vi "EOL CAN_Get Key C70.vi"(11 "Seed message":u8[](array[numeric])=[6, 103, 1, 36, 34, 32, 31, 0] format="%x") -> (3 "Key":u32[](array[numeric]) format="%x")   [LabVIEW 2018]
panel:
  out "(hi.lo)":u32
  out "Seed":u32[](array[numeric])=[6, 103, 1, 36, 34, 32, 31, 0] format="%x"
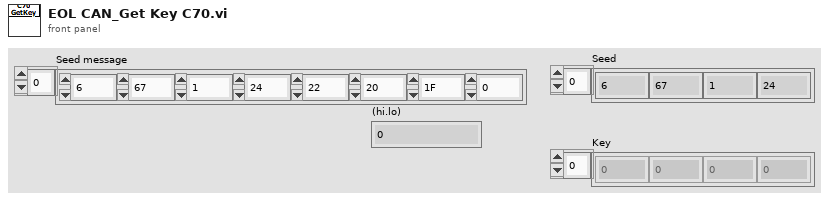
[diagram p1: front panel]
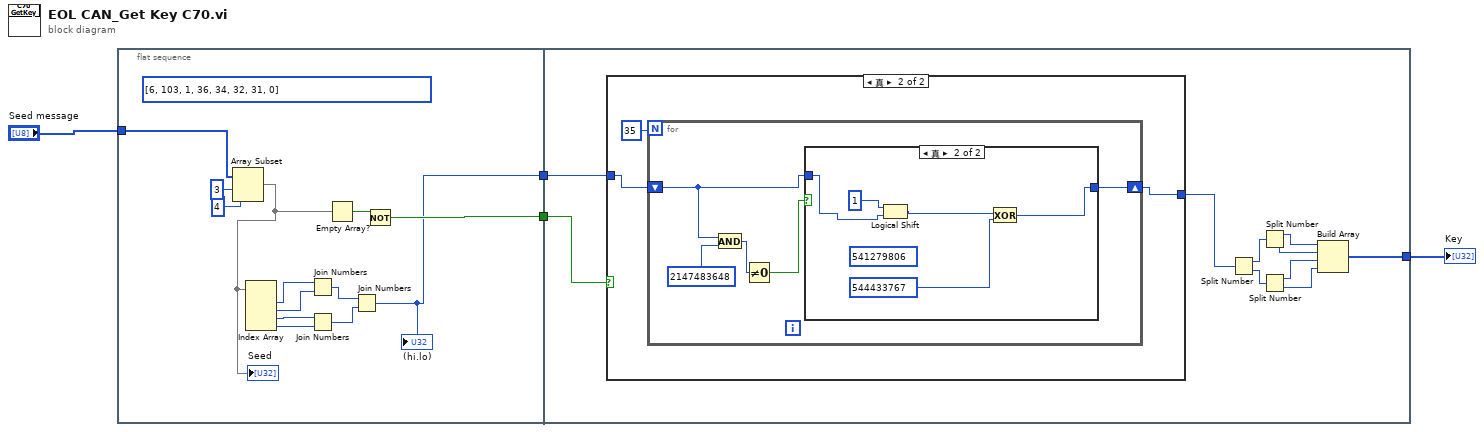
[diagram p0: block diagram]
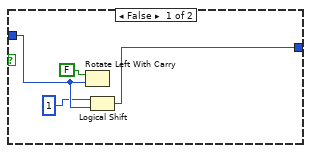
[diagram p3: hidden frame]
diagram:
  n1 = flat-sequence {
    tunnel: [w14] -> w4
    tunnel: [w7] -> w3
    tunnel: "Seed message" -> [w5]
    tunnel: w4 -> [w27]
    tunnel: w3 -> [w26]
    tunnel: [w18] -> w2
    frame #0 {
      (unwired) u8[] [6, 103, 1, 36, 34, 32, 31, 0] ("Transmit Data 2")
      n2 = Array Subset(array=w5, index=3 ("索引"), length=4 ("长度")) -> (w6:u8[])
      "Seed" <- w6
      n3 = Index Array(array=w6) -> (element #1=w13:u8, element #2=w12:u8, element #3=w11:u8, element #4=w10:u8)  [unwired: 4 in]
      n4 = Join Numbers(hi=w13, lo=w12) -> ((hi.lo)=w9:u16)
      n5 = Join Numbers(hi=w11, lo=w10) -> ((hi.lo)=w8:u16)
      n6 = Empty Array?(array=w6) -> (empty?=w15:bool)
      n7 = Join Numbers(hi=w9, lo=w8) -> ((hi.lo)=w7:u32)
      "(hi.lo)" <- w7
      n8 = Not(x=w15) -> (.not. x?=w14:bool)
    }
    frame #1 {
      n9 = case shown="真" w27 {
        tunnel: w26 -> [w28 w30]
        tunnel: [w28 w29] -> w25
        frame False {
        }
        frame True {
          n10 = for {
            N: 35 -> [_]
            shift-right: [w36] -> w29
            shift-left: w30 -> [w34]
            n11 = And(x=w34, y=u32 2147483648) -> (x .and. y?=w33:u32)
            n12 = Not Equal To 0?(x=w33) -> (x != 0?=w32:bool)
            n13 = case shown="真" w32 {
              tunnel: w34 -> [w38 w44]
              tunnel: [w39 w45] -> w36
              frame False {
                n14 = Rotate Left With Carry(2:w38, 3:FALSE ("进位")) -> ()  [unwired: 2 out]
                n15 = Logical Shift(y=u32 1 ("x"), x=w38) -> (x << y=w39:u32)
              }
              frame True {
                (unwired) u32 541279806
                n16 = Logical Shift(y=u32 1 ("x"), x=w44) -> (x << y=w43:u32)
                n17 = Exclusive Or(1:u32 544433767, 2:w43) -> (0:w45:u32)
              }
            }
          }
        }
      }
      n18 = Split Number(x=w25) -> (hi(x)=w23:u16, lo(x)=w24:u16)
      n19 = Split Number(x=w23) -> (hi(x)=w22:u8, lo(x)=w21:u8)
      n20 = Split Number(x=w24) -> (hi(x)=w20:u8, lo(x)=w19:u8)
      n21 = Build Array(w22, w21, w20, w19) -> (w18:u8[])
    }
  }
  "Key" <- w2
